vi "Receive Message.vi"(6 "priority":i32, 10 "IMediatorBusMonitor in":refnum<class "IMediatorBusMonitor.lvclass">, 11 "Message in":refnum<class "Message.lvclass">) -> (0 "error out":errorcluster, 2 "Actor out":refnum<class "Actor.lvclass">)   [LabVIEW 2017, in "IMediator.lvlib" / "IMediatorBusMonitor.lvclass"]
doc: "This VI should be overriden ONLY if you are creating a proxy actor for remote transmission. If you are, override this VI to transmit the received message to a new destination, maintaining the given priority."
uses:
  IMediatorBusMonitor.lvclass
  <vilib>/ActorFramework/Message/Message.lvclass
  <vilib>/ActorFramework/Actor/Actor.lvclass
  C:/Program Files (x86)/National Instruments/LabVIEW 2017/vi.lib/ActorFramework/Actor/Actor.lvclass
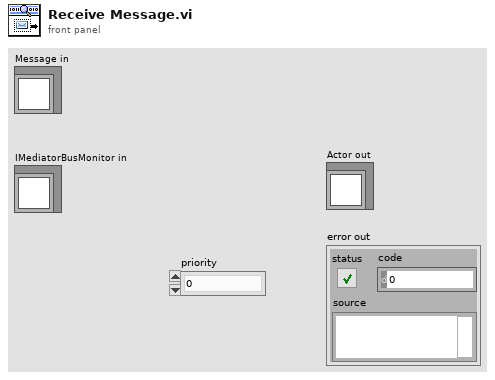
[diagram p1: front panel]
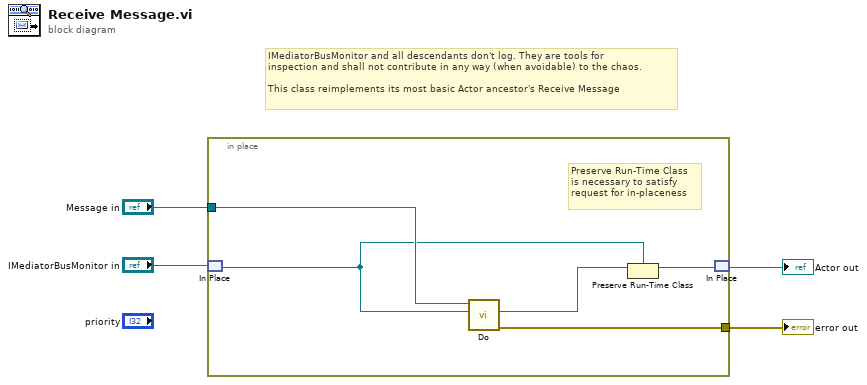
[diagram p0: block diagram]
diagram:
  # "IMediatorBusMonitor and all descendants don't log. They are tools for\ninspection and shall not contribute in any way (when avoidable) to the chaos.\n\nThis class reimplements its most basic Actor ancestor's Receive Message"
  n1 = in-place {
    in-place-border: [w9] -> w2
    in-place-border: "Message in" -> [w8]
    # "Preserve Run-Time Class\nis necessary to satisfy\nrequest for in-placeness"
    n2 = in-place-match #1("IMediatorBusMonitor in") -> (w5:refnum<class "IMediatorBusMonitor.lvclass">)
    n3 = call-dynamic "Do.vi"("Actor in"=w5, "Message"=w8) -> ("error out"=w9:errorcluster, "Actor out"=w7:refnum<class "Actor.lvclass">)  [unwired: 8 in]
    n4 = Preserve Run-Time Class(object in=w7, 2:w5) -> (object out=w6:refnum<class "IMediatorBusMonitor.lvclass">)  [unwired: 1 in, 1 out]
    n5 = in-place-match #1(w6) -> (→"Actor out":refnum<class "IMediatorBusMonitor.lvclass">)
  }
  "error out" <- w2
